vi "DAQNavi Read (Analog 2D U32 NChan NSamp).vi"(8 "error in (no error)":errorcluster, 9 "number of samples per channel to read":u32=1000, 10 "timeout":dbl=10.0 format="%0.2f", 11 "task in":i32) -> (0 "error out":errorcluster, 1 "markBuf":cluster{"Data Index":i64, "Src Id":i64}[](array[cluster]), 2 "data":u32[][](array[numeric]), 3 "task out":i32)   [LabVIEW 2020]
uses:
  DAQNavi_LV.dll
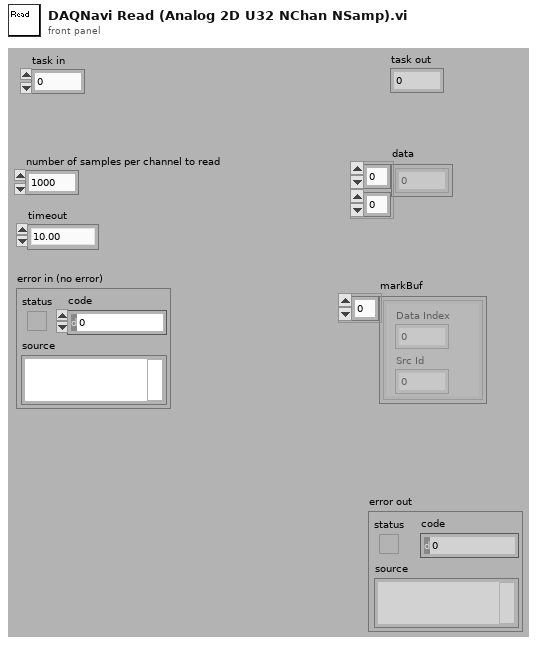
[diagram p1: front panel]
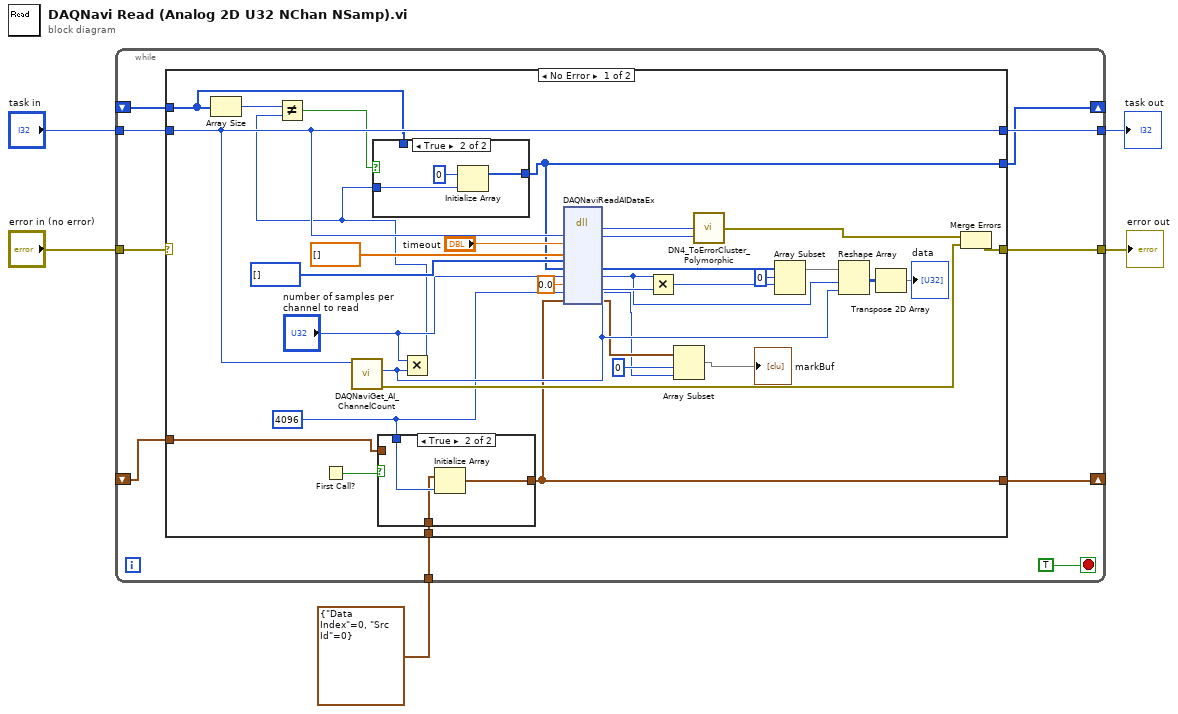
[diagram p0: block diagram]
diagram:
  n1 = while {
    tunnel: "task in" -> [w15]
    tunnel: "error in (no error)" -> [w14]
    tunnel: [w13] -> w3
    tunnel: [w12] -> w2
    shift-right: [w10] -> _
    shift-left: _ -> [w9]
    tunnel: cluster{"Data Index":i64, "Src Id":i64} {"Data Index"=0, "Src Id"=0} -> [w8]
    shift-right: [w7] -> _
    shift-left: _ -> [w6]
    stop <- TRUE stop-if-true
    n2 = case shown="No Error" w14 {
      selector: w14 -> [_ w59]
      tunnel: w15 -> [w42 w60]
      tunnel: [w42 w60] -> w13
      tunnel: [w41 w59] -> w12
      tunnel: [w26 w57] -> w10
      tunnel: w9 -> [w27 w57]
      tunnel: w8 -> [w22 _]
      tunnel: [w20 w58] -> w7
      tunnel: w6 -> [w21 w58]
      frame No Error {
        w23 = 4096
        n3 = Array Size(array=w27) -> (size(s)=w30:i32)
        n4 = First Call?() -> (First Call?: T/F=w24:bool)
        n5 = call "DAQNaviGet_AI_ChannelCount.vi"("task in"=w42) -> ("error out"=w39:errorcluster, "channel count"=w34:i32)  [unwired: 1 in, 8 out]
        n6 = case shown="True" w24 {
          tunnel: w23 -> [_ w52]
          tunnel: w22 -> [_ w51]
          tunnel: [w49 w50] -> w20
          tunnel: w21 -> [w49 _]
          frame False {
          }
          frame True {
            n7 = Initialize Array(w51, w52) -> (w50:cluster{"Data Index":i64, "Src Id":i64}[])
          }
        }
        n8 = Multiply(x="number of samples per channel to read", y=w34) -> (x*y=w28:u32)
        n9 = Not Equal?(x=w30, y=w28) -> (x != y?=w29:bool)
        n10 = case shown="True" w29 {
          tunnel: [w53 w55] -> w26
          tunnel: w28 -> [_ w54]
          tunnel: w27 -> [w53 _]
          frame False {
          }
          frame True {
            n11 = Initialize Array(u32 0 ("element"), w54) -> (w55:u32[])
          }
        }
        n12 = dll-call lib="DAQNavi_LV.dll" fn="DAQNaviReadAIDataEx"("taskID"=w42, "timeout"="timeout", "scaledData"=dbl[] [], "rawData16"=u16[] [] ("rawData32"), "rawData32"=w26, "samples"="number of samples per channel to read", "startTime"=0.0, "markCount"=w23, "markBuf"=w20) -> ("return type"=w46:i32, "taskID"=w31:i32, "rawData32"=w44:u32[], "samples"=w33:u32, "markCount"=w17:i32, "markBuf"=w19:cluster{"Data Index":i64, "Src Id":i64}[])  [unwired: 4 in, 5 out]
        n13 = Multiply(x=w33, y=w34) -> (x*y=w35:u32)
        n14 = Array Subset(array=w19, index=0, length=w17) -> (→"markBuf":cluster{"Data Index":i64, "Src Id":i64}[])
        n15 = call "DN4_ToErrorCluster_Polymorphic.vi"("task id"=w31, "error code"=w46) -> ("error out"=w40:errorcluster)  [unwired: 3 out]
        n16 = Array Subset(array=w44, index=0, length=w35) -> (w38:u32[])
        n17 = Reshape Array(w38, w33, w34) -> (w37:u32[][])
        n18 = Transpose 2D Array(2D array=w37) -> (transposed array=→"data":u32[][])
        n19 = Merge Errors(w40, w39) -> (w41:errorcluster)
      }
      frame Error {
      }
    }
  }
  "task out" <- w3
  "error out" <- w2
